vi "Init.vi"(10 "Info Synapses":T2(array[cluster])=[{"Conv %"=4.0, "Synapse"=enum."MF to GC", "Weight Gain"=1.0}, {"Conv %"=4.0, "Synapse"=enum."GO to GC", "Weight Gain"=-0.3}, {"Conv %"=0.4, "Synapse"=enum."GC to GO", "Weight Gain"=1.0}, {"Conv %"=0.5, "Synapse"=enum."MF to GO", "Weight Gain"=1.0}, {"Conv %"=0.5, "Synapse"=enum."GC to PC", "Weight Gain"=2.0}, {"Conv %"=0.1, "Synapse"=enum."GC to BA", "Weight Gain"=2.0}, {"Conv %"=0.01, "Synapse"=enum."PC to BA", "Weight Gain"=-0.1}, {"Conv %"=0.4, "Synapse"=enum."BA to PC", "Weight Gain"=-0.1}, {"Conv %"=0.1, "Synapse"=enum."BA to GO", "Weight Gain"=-0.5}], 11 "Grid in":refnum<class "Grid.lvclass">=refnum) -> (2 "Grid out":refnum<class "Grid.lvclass">, 3 "Synapses out":refnum<class "Synapses.lvclass">)   [LabVIEW 2013, in "Synapses.lvclass"]
doc: "This Vi initialize the vectors required to store the synaptic connections configured. It calculates the divergenece ratios as Npost*Conv/Npre"
uses:
  Synapses.lvclass
  Controls/Type of Synapses.ctl
  Cube/Grid.lvclass
  Neuron/Neuron.lvclass
  Cube/Grid.lvclass/Grid.ctl
  Controls/Synapses.ctl
  Neuron/Neuron.lvclass/Neuron.ctl
  Synapses.lvclass/Synapses.ctl
  Neuron/Get Neuron Properties.vi
panel:
  out "Conv":i32[](array[numeric])=[4, 4, 240, 20, 300, 60, 1, 24, 6]
  out "Div":i32[](array[numeric])=[60, 600, 2, 2, 1, 6, 60, 1, 1]
  out "size(s)":i32=9
  # "Conv% with respect to the No of Presynaptic Neurons"
  # "Weight Gain with respect to the No of Presynaptic Neurons"
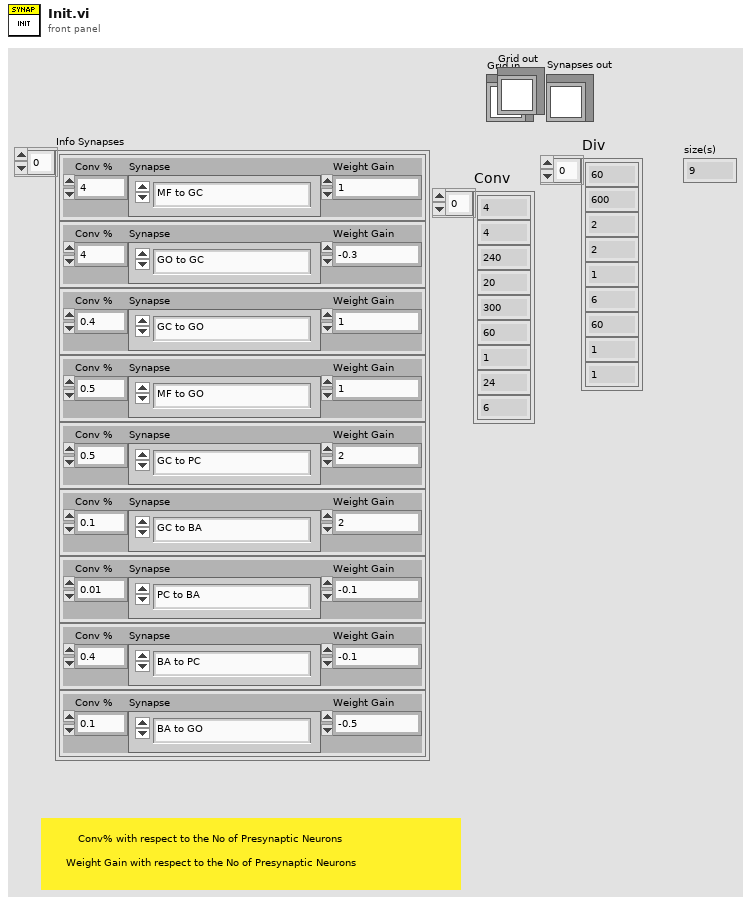
[diagram p1: front panel]
types:
  T1 = typedef "Type of Synapses.ctl" = enum16{"MF to GC", "GO to GC", "GC to GO", "MF to GO", "GC to PC", "GC to BA", "PC to BA", "BA to PC", "BA to GO"}
  T2 = cluster{"Conv %":dbl, "Synapse":T1, "Weight Gain":dbl}[]
  T3 = typedef "Synapses.ctl" = cluster{"Synapse":T1, "Pre_List":i32[][], "Post_List":i32[][], "Weight gain":dbl}
  T4 = typedef "Type of Neuron.ctl" = enum16{"MF", "BA", "GO", "GC", "PC", "LU", "Glia (Dummy)"}
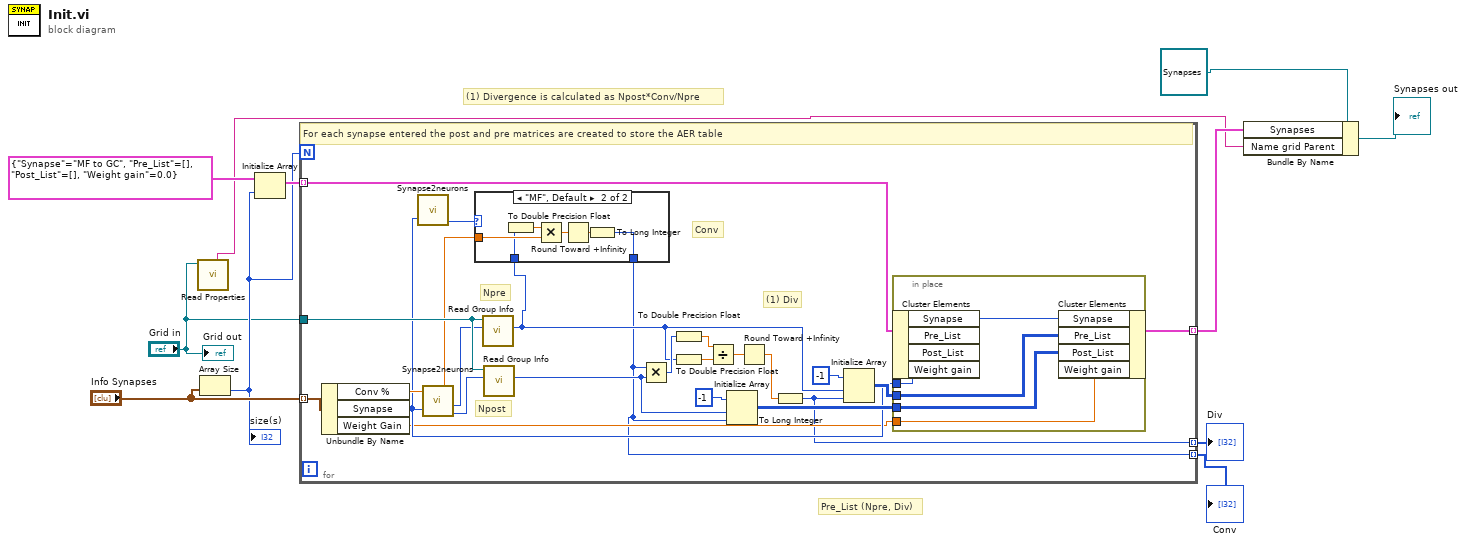
[diagram p0: block diagram]
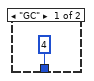
[diagram p2: hidden frame]
diagram:
  # "Pre_List (Npre, Div)"
  # "(1) Divergence is calculated as Npost*Conv/Npre"
  n1 = call "Read Properties.vi"("Grid in"="Grid in") -> ("Name XML File"=w3:string)  [unwired: 3 in, 7 out]
  n2 = Array Size(array="Info Synapses") -> (size(s)=w5:i32)
  "size(s)" <- w5
  n3 = Initialize Array(T3 {"Synapse"=enum."MF to GC", "Pre_List"=[], "Post_List"=[], "Weight gain"=0.0} ("Synapses"), w5) -> (w7:T3[])
  n4 = for {
    N: w5 -> [_]
    tunnel: "Grid in" -> [w34]
    tunnel: "Info Synapses" -> [w26] mode=indexing
    tunnel: w7 -> [w19] mode=indexing
    tunnel: [w21] -> w6 mode=indexing
    tunnel: [w13] -> w2 mode=indexing
    tunnel: [w12] -> w1 mode=indexing
    # "Conv"
    # "(1) Div"
    # "Npost"
    # "Npre"
    # "For each synapse entered the post and pre matrices are created to store the AER table"
    n5 = Unbundle By Name(w26) -> ("Conv %"=w18:dbl, "Synapse"=w15:T1, "Weight Gain"=w14:dbl)
    n6 = call "Synapse2neurons.vi"("Synapse"=w15) -> ("Post Neuron"=w17:T4)  [unwired: 4 in, 1 out]
    n7 = call "Synapse2neurons.vi"("Synapse"=w15) -> ("Post Neuron"=w32:T4, "Pre Neuron"=w33:T4)  [unwired: 4 in]
    n8 = call "Read Group Info.vi"("Neuron Type"=w33, "Grid in"=w34) -> ("N"=w16:i32)  [unwired: 7 in, 2 out]
    n9 = case shown="\"MF\", Default" w17 {
      tunnel: [4 w38] -> w12
      tunnel: w18 -> [_ w37]
      tunnel: w16 -> [_ w36]
      frame "GC" {
      }
      frame "MF", Default {
        n10 = To Double Precision Float(number=w36) -> (double precision float=w41:dbl)
        n11 = Multiply(x=w41, y=w37) -> (x*y=w39:dbl)
        n12 = Round Toward +Infinity(x=w39) -> (ceil(x): smallest int >= x=w40:dbl)
        n13 = To Long Integer(number=w40) -> (32bit integer=w38:i32)
      }
    }
    n14 = call "Read Group Info.vi"("Neuron Type"=w32, "Grid in"=w34) -> ("N"=w20:i32)  [unwired: 7 in, 2 out]
    n15 = Multiply(x=w12, y=w20) -> (x*y=w31:i32)
    n16 = To Double Precision Float(number=w31) -> (double precision float=w27:dbl)
    n17 = To Double Precision Float(number=w16) -> (double precision float=w28:dbl)
    n18 = Divide(x=w27, y=w28) -> (x/y=w30:dbl)
    n19 = Initialize Array(-1 ("x*y"), w20, w12) -> (w22:i32[][])
    n20 = Round Toward +Infinity(x=w30) -> (ceil(x): smallest int >= x=w29:dbl)
    n21 = To Long Integer(number=w29) -> (32bit integer=w13:i32)
    n22 = Initialize Array(-1 ("x*y"), w16, w13) -> (w23:i32[][])
    n23 = in-place {
      in-place-border: w23 -> [w45]
      in-place-border: w22 -> [w44]
      in-place-border: w15 -> [w43]
      in-place-border: w14 -> [w42]
      n24 = in-place-cluster #1(w19) -> ()  [unwired: 4 out]
      n25 = in-place-cluster #1("Synapse"=w43, "Pre_List"=w45, "Post_List"=w44, "Weight gain"=w42) -> (w21:T3)
    }
  }
  "Div" <- w2
  "Conv" <- w1
  n26 = Bundle By Name(cluster=refnum<class "Synapses.lvclass"> refnum ("Synapses in"), "Synapses"=w6, "Name grid Parent"=w3) -> (→"Synapses out":refnum<class "Synapses.lvclass">)
  "Grid out" <- "Grid in"
